vi "Stopv2.vi"   [LabVIEW 2015]
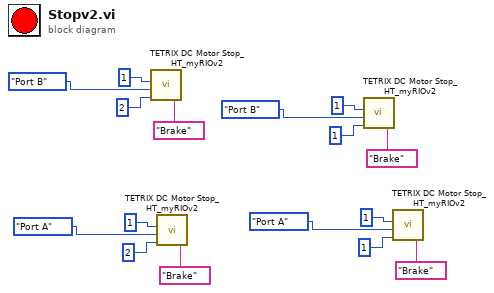
[diagram p0: block diagram]
diagram:
  n1 = call "TETRIX DC Motor Stop_HT_myRIOv2.vi"("Stop (Brake or Coast)"="Brake", "Motor Channel: (1 or 2)"=u8 2, "Port"=enum16{"Port A", "Port B", ""}."Port B", "Controller Daisy Chain Position: 1 - 4"=u8 1) -> ()  [unwired: 1 in, 1 out]
  n2 = call "TETRIX DC Motor Stop_HT_myRIOv2.vi"("Stop (Brake or Coast)"="Brake", "Motor Channel: (1 or 2)"=u8 2, "Port"=enum16{"Port A", "Port B", ""}."Port A", "Controller Daisy Chain Position: 1 - 4"=u8 1) -> ()  [unwired: 1 in, 1 out]
  n3 = call "TETRIX DC Motor Stop_HT_myRIOv2.vi"("Stop (Brake or Coast)"="Brake", "Motor Channel: (1 or 2)"=u8 1, "Port"=enum16{"Port A", "Port B", ""}."Port B", "Controller Daisy Chain Position: 1 - 4"=u8 1) -> ()  [unwired: 1 in, 1 out]
  n4 = call "TETRIX DC Motor Stop_HT_myRIOv2.vi"("Stop (Brake or Coast)"="Brake", "Motor Channel: (1 or 2)"=u8 1, "Port"=enum16{"Port A", "Port B", ""}."Port A", "Controller Daisy Chain Position: 1 - 4"=u8 1) -> ()  [unwired: 1 in, 1 out]
